vi "Table Select Single Row.vi"(9 "Row Location":T1, 11 "Table Ref In":refnum<vi>) -> (3 "Table Ref Out":refnum<vi>)   [LabVIEW 2024]
uses:
  <vilib>/Utility/miscctls.llb/LVRowAndColumnTypeDef.ctl
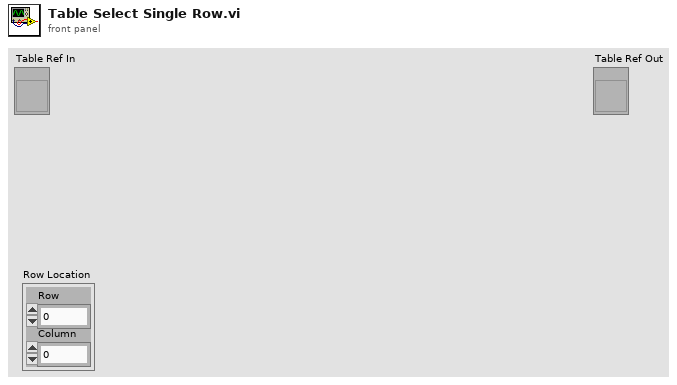
[diagram p1: front panel]
types:
  T1 = typedef "LVRowAndColumnTypeDef.ctl" = cluster{"Row":i32, "Column":i32}
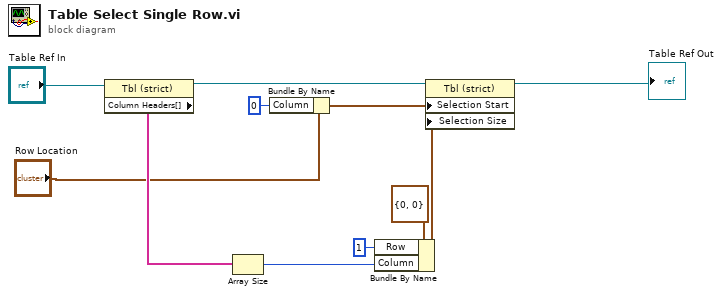
[diagram p0: block diagram]
diagram:
  n1 = property class="Tbl (strict)"(reference="Table Ref In") -> (reference out=w10:refnum<vi>, "Column Headers[]"=w9:string[])  [unwired: 1 in, 1 out]
  n2 = Array Size(array=w9) -> (size(s)=w5:i32)
  n3 = Bundle By Name(cluster="Row Location", "Column"=0) -> (w1:T1)
  n4 = Bundle By Name(cluster=T1 {"Row"=0, "Column"=0} ("Selection Size"), "Row"=1, "Column"=w5) -> (w6:T1)
  n5 = property class="Tbl (strict)"(reference=w10, "Selection Start"=w1, "Selection Size"=w6) -> (reference out=→"Table Ref Out":refnum<vi>)  [unwired: 1 in, 1 out]
